vi "Assert Brower Controller.vi"() -> ()   [LabVIEW 2015, in "BrowerController.lvclass"]
uses:
  BrowerController.lvclass
  Type Definition/Brower UI Refs.ctl
  Models/BrowerTree/BrowerTree.lvclass
  Models/BrowerBuilder/ProjectBuilder/ProjectBuilder.lvclass
  Models/BrowerComponent/BrowerComposite/BrowerComposite.lvclass
  BrowerController.lvclass/BrowerController.ctl
panel:
  in  "Tree":string(tree)
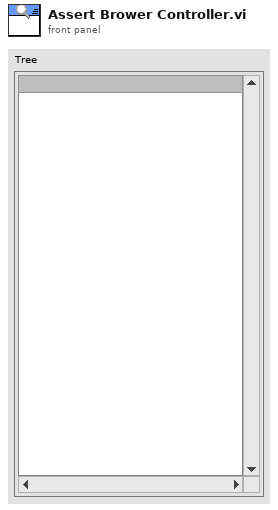
[diagram p1: front panel]
types:
  T1 = typedef "BrowerController.lvclass/Brower UI Refs.ctl" = cluster{"BrowerTree Ref":refnum<vi>, "BrowerMenu Selection(\"\")":refnum<vi>, "VI Refnum":refnum<vi>}
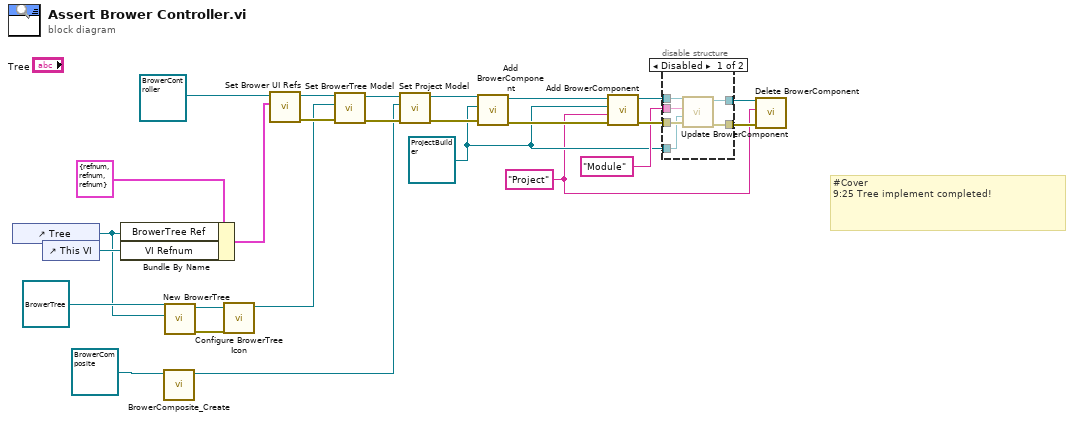
[diagram p0: block diagram]
diagram:
  w1 = "Project" ("Parent Tag(\"\")")
  w4 = refnum<class "ProjectBuilder.lvclass"> refnum ("ProjectBuilder")
  # "#Cover \n9:25 Tree implement completed!"
  n1 = control-ref of="Tree"() -> (w19:refnum<vi>)
  n2 = control-ref of="This VI"() -> (w24:refnum<vi>)
  n3 = Bundle By Name(cluster=T1 {"BrowerTree Ref"=refnum, "BrowerMenu Selection(\"\")"=refnum, "VI Refnum"=refnum} ("Brower UI Refs"), "BrowerTree Ref"=w19, "VI Refnum"=w24) -> (w23:T1)
  n4 = call "BrowerComposite_Create.vi"("reference in"=refnum<class "BrowerComposite.lvclass"> refnum ("BrowerComposite")) -> ("reference out"=w12:refnum<class "BrowerComposite.lvclass">)  [unwired: 9 in, 1 out]
  n5 = call "New BrowerTree.vi"("Tree Refnum"=w19, "BrowerTree in"=refnum<class "BrowerTree.lvclass"> refnum ("BrowerTree.lvclass")) -> ("error out"=w17:errorcluster, "BrowerTree out"=w18:refnum<class "BrowerTree.lvclass">)  [unwired: 8 in]
  n6 = call "Configure BrowerTree Icon.vi"("error in (no error)"=w17, "BrowerTree in"=w18) -> ("BrowerTree out"=w16:refnum<class "BrowerTree.lvclass">)  [unwired: 8 in, 1 out]
  n7 = call "Set Brower UI Refs.vi"("Brower UI Refs"=w23, "BrowerController in"=refnum<class "BrowerController.lvclass"> refnum) -> ("error out"=w21:errorcluster, "BrowerController out"=w22:refnum<class "BrowerController.lvclass">)  [unwired: 8 in]
  n8 = call "Set BrowerTree Model.vi"("error in (no error)"=w21, "BrowerTree.lvclass"=w16, "BrowerController in"=w22) -> ("error out"=w13:errorcluster, "BrowerController out"=w14:refnum<class "BrowerController.lvclass">)  [unwired: 7 in]
  n9 = call "Set Project Model.vi"("error in (no error)"=w13, "Project.lvclass"=w12, "BrowerController in"=w14) -> ("error out"=w10:errorcluster, "BrowerController out"=w11:refnum<class "BrowerController.lvclass">)  [unwired: 7 in]
  n10 = call "Add BrowerComponent.vi"("error in (no error)"=w10, "Builder"=w4, "BrowerController in"=w11) -> ("error out"=w8:errorcluster, "BrowerController out"=w9:refnum<class "BrowerController.lvclass">)  [unwired: 7 in]
  n11 = call "Add BrowerComponent.vi"("error in (no error)"=w8, "Parent Tag(\"\")"=w1, "Builder"=w4, "BrowerController in"=w9) -> ("error out"=w6:errorcluster, "BrowerController out"=w7:refnum<class "BrowerController.lvclass">)  [unwired: 6 in]
  n12 = disable-structure shown="Disabled" {
    disable-tunnel: w7 -> [w32 w34]
    disable-tunnel: w6 -> [w31 w33]
    disable-tunnel: "Module" ("BrowerComponentID(\"\")") -> [w30 _]
    disable-tunnel: w4 -> [w29 _]
    disable-tunnel: [w28 w34] -> w3
    disable-tunnel: [w27 w33] -> w2
    frame Disabled {
      n13 = call "Update BrowerComponent.vi"("error in (no error)"=w31, "AbstractBuilder"=w29, "BrowerComponentID(\"\")"=w30, "BrowerController in"=w32) -> ("error out"=w27:errorcluster, "BrowerController out"=w28:refnum<class "BrowerController.lvclass">)  [unwired: 6 in]
    }
    frame Enabled {
    }
  }
  n14 = call "Delete BrowerComponent.vi"("error in (no error)"=w2, "BrowerComponentID(\"\")"=w1, "BrowerController in"=w3) -> ()  [unwired: 7 in, 2 out]
